vi "Cycle_Diag_Table_Read_TL24.vi"(7 "ERD Data In":T3[](array[typedef]) {"ERD Number" format="%.0x"}, 11 "error in (no error)":errorcluster) -> (2 "Cycle Buffer Status":T2, 3 "Diag Cycle String Out":string[][](array[string]), 8 "Cycle  Diag Array Out":T1[](array[typedef]), 15 "error out":errorcluster)   [LabVIEW 2016]
uses:
  Common/LabVIEW GEA2 Toolkit/LabVIEW_GEA2_Toolkit.lvlibp/type defs/ERD Read Data Out.ctl
  type defs/Cycle_Diag_Buffer_Status.ctl
  type defs/Cycle_Diag.ctl
  Common/LabVIEW GEA2 Toolkit/LabVIEW_GEA2_Toolkit.lvlibp
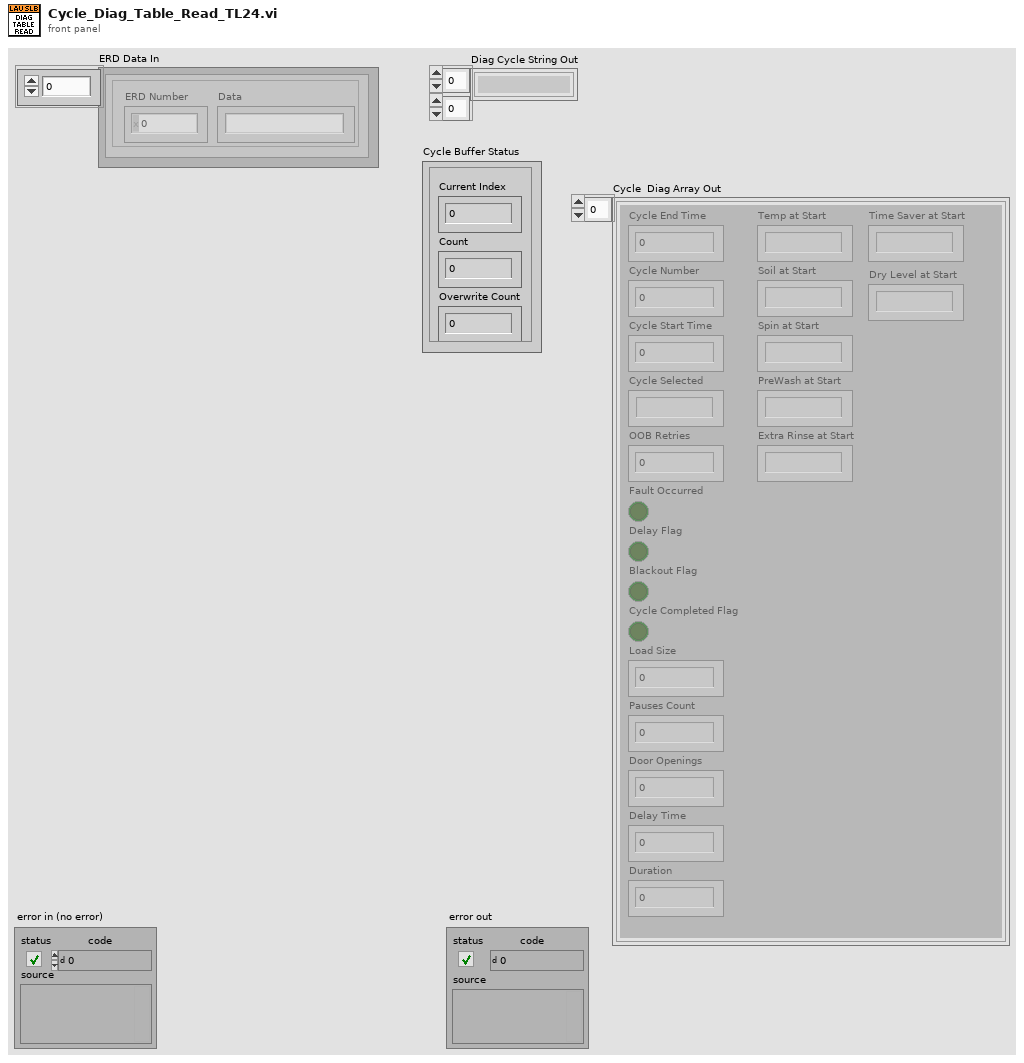
[diagram p1: front panel]
types:
  T1 = typedef "Cycle_Diag.ctl" = cluster{"Cycle End Time":u32, "Cycle Number":u32, "Cycle Start Time":u32, "OOB Retries":u8, "Temp at Start":string, "Soil at Start":string, "PreWash at Start":string, "Extra Rinse at Start":string, "Pauses Count":u8, "Fault Occurred":bool, "Delay Flag":bool, "Blackout Flag":bool, "Cycle Completed Flag":bool, "Time Saver at Start":string, "Load Size":u8, "Door Openings":u8, "Cycle Selected":string, "Spin at Start":string, "Delay Time":u16, "Duration":dbl, "Dry Level at Start":string}
  T2 = typedef "Cycle_Diag_Buffer_Status.ctl" = cluster{"Current Index":u16, "Count":u16, "Overwrite Count":u16}
  T3 = typedef "LabVIEW_GEA2_Toolkit.lvlibp/ERD Read Data Out.ctl" = cluster{"ERD Number":u16, "Data":string}
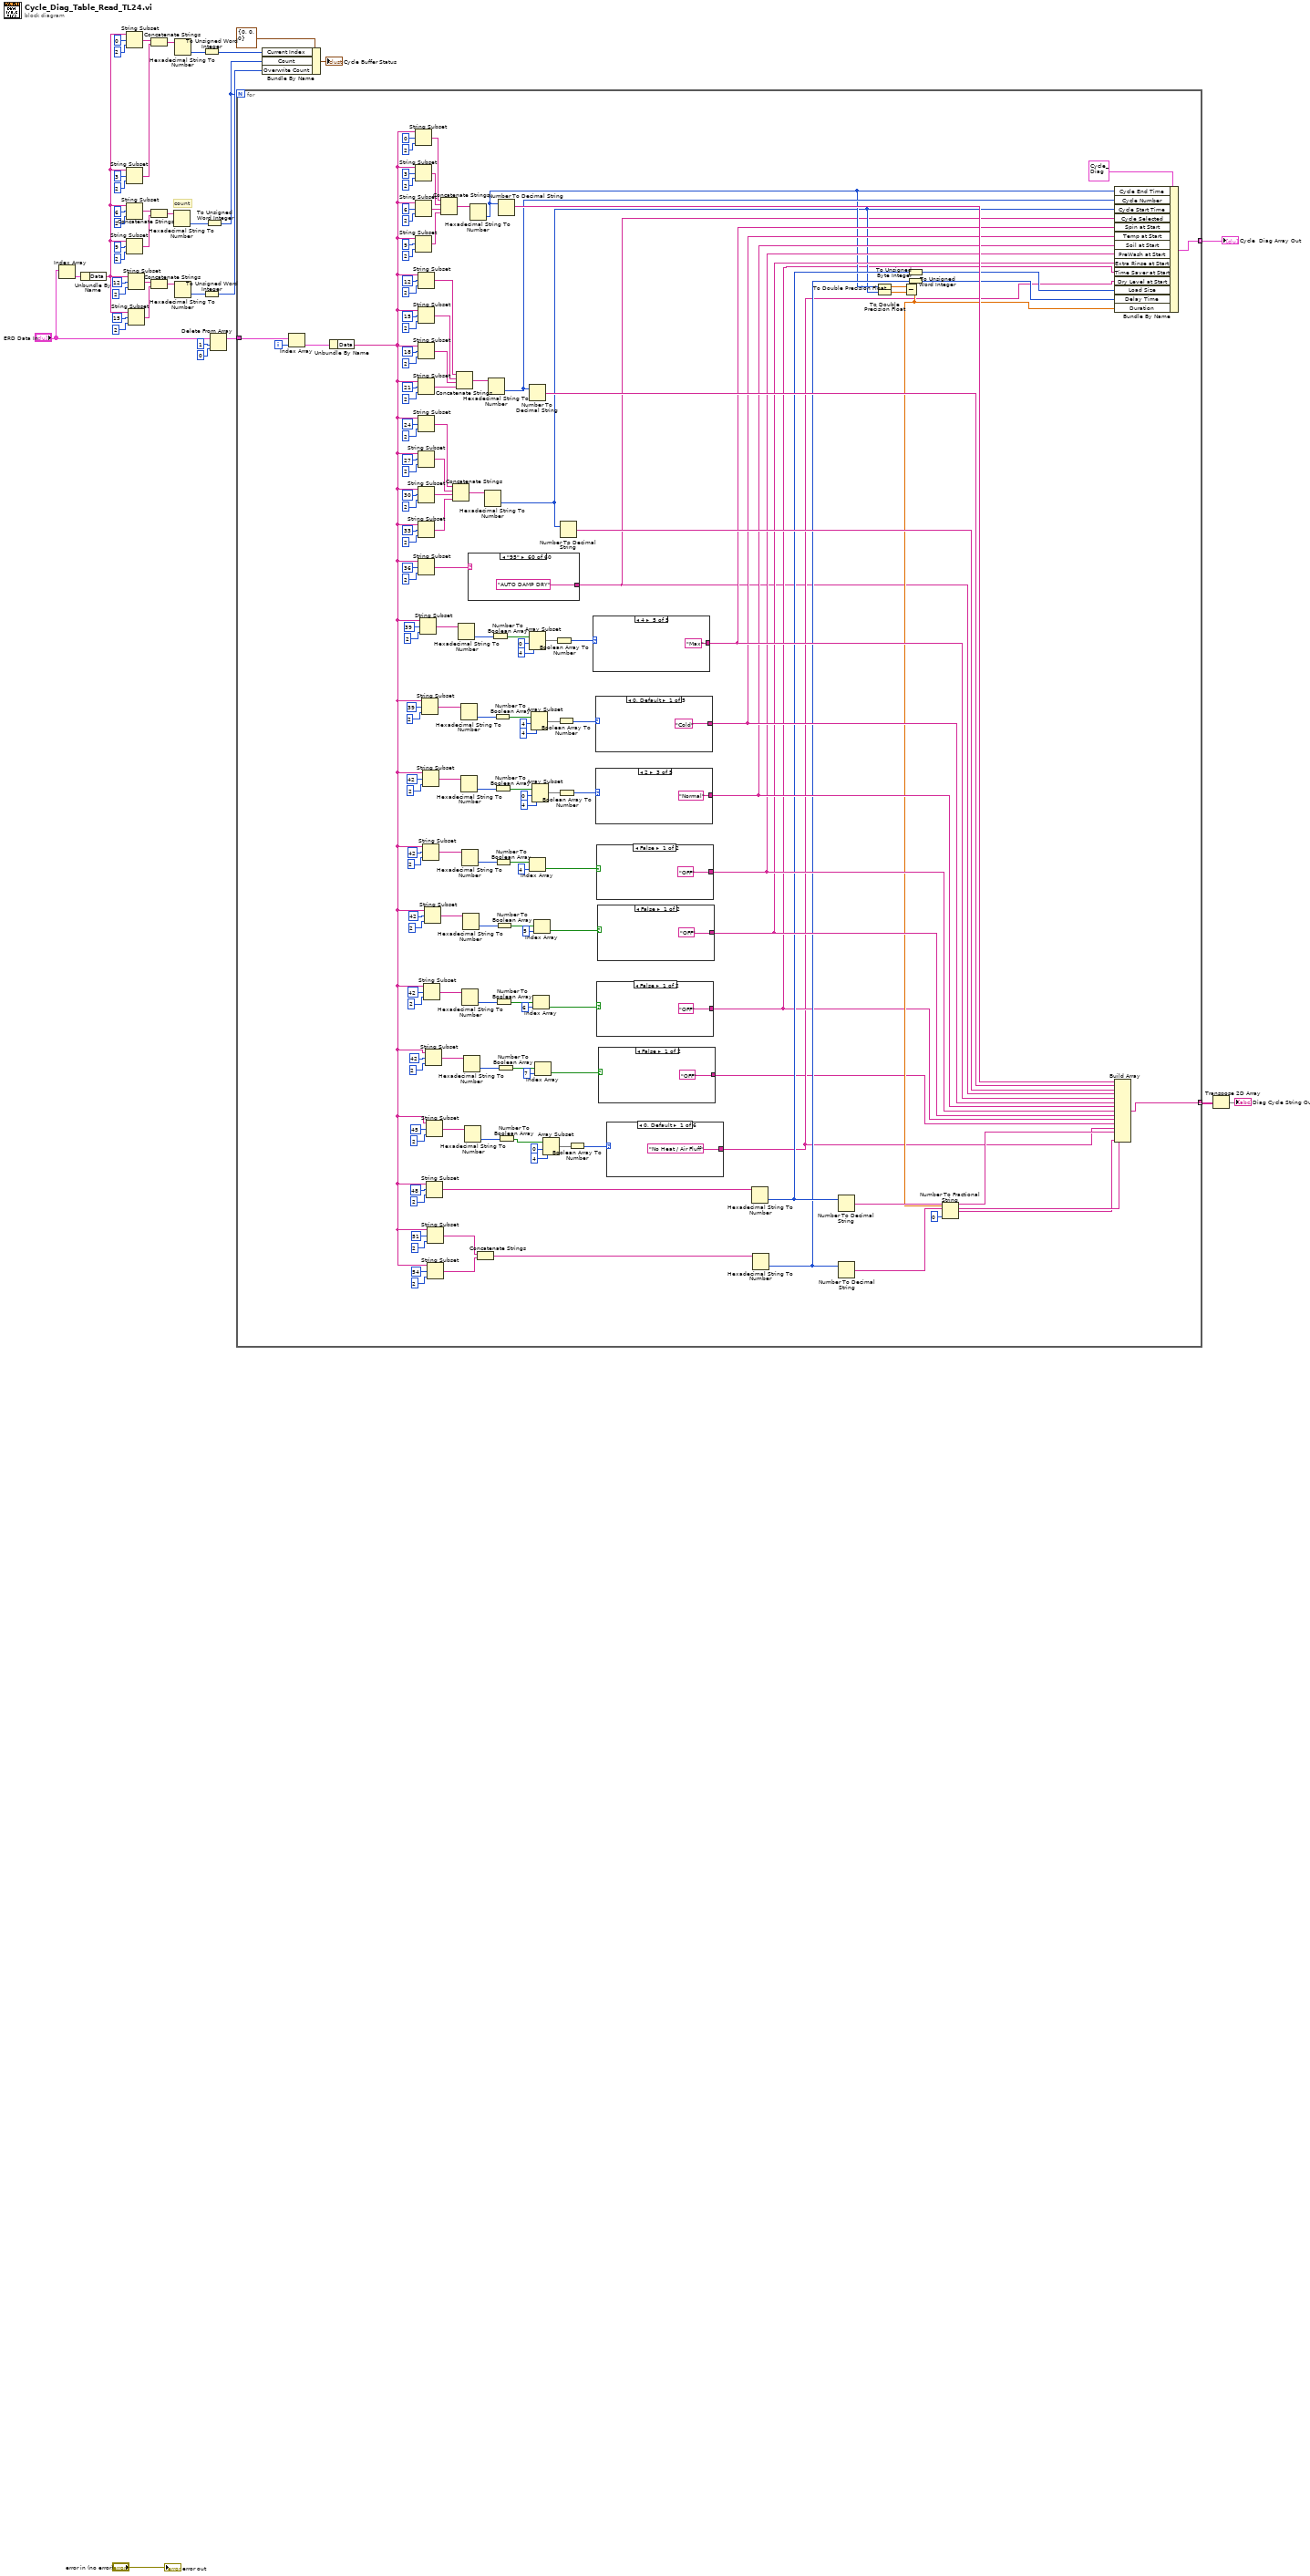
[diagram p0: block diagram]
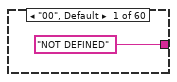
[diagram p2: hidden frame]
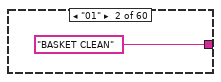
[diagram p3: hidden frame]
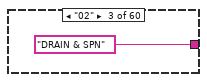
[diagram p4: hidden frame]
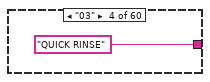
[diagram p5: hidden frame]
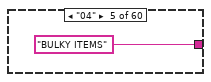
[diagram p6: hidden frame]
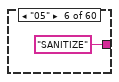
[diagram p7: hidden frame]
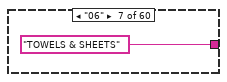
[diagram p8: hidden frame]
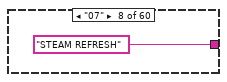
[diagram p9: hidden frame]
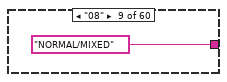
[diagram p10: hidden frame]
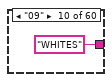
[diagram p11: hidden frame]
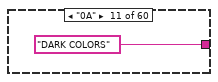
[diagram p12: hidden frame]
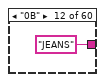
[diagram p13: hidden frame]
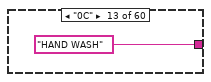
[diagram p14: hidden frame]
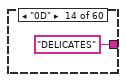
[diagram p15: hidden frame]
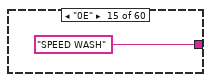
[diagram p16: hidden frame]
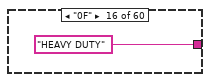
[diagram p17: hidden frame]
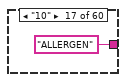
[diagram p18: hidden frame]
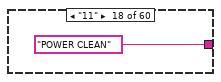
[diagram p19: hidden frame]
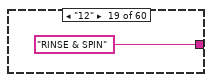
[diagram p20: hidden frame]
diagram:
  # "count"
  n1 = Index Array(array="ERD Data In") -> (element=w32:T3)  [unwired: 1 in]
  n2 = Unbundle By Name(w32) -> ("Data"=w12:string)
  n3 = String Subset(string=w12, offset (0)=0, length (rest)=2 ("length (rest)")) -> (substring=w21:string)
  n4 = String Subset(string=w12, offset (0)=3, length (rest)=2 ("length (rest)")) -> (substring=w22:string)
  n5 = String Subset(string=w12, offset (0)=6, length (rest)=2 ("length (rest)")) -> (substring=w36:string)
  n6 = String Subset(string=w12, offset (0)=9, length (rest)=2 ("length (rest)")) -> (substring=w35:string)
  n7 = String Subset(string=w12, offset (0)=12, length (rest)=2 ("length (rest)")) -> (substring=w23:string)
  n8 = String Subset(string=w12, offset (0)=15, length (rest)=2 ("length (rest)")) -> (substring=w24:string)
  n9 = Concatenate Strings(w21, w22) -> (w25:string)
  n10 = Concatenate Strings(w36, w35) -> (w34:string)
  n11 = Concatenate Strings(w23, w24) -> (w26:string)
  n12 = Hexadecimal String To Number(string=w34) -> (number=w33:u32)  [unwired: 2 in, 1 out]
  n13 = Hexadecimal String To Number(string=w25) -> (number=w27:u32)  [unwired: 2 in, 1 out]
  n14 = Hexadecimal String To Number(string=w26) -> (number=w28:u32)  [unwired: 2 in, 1 out]
  n15 = To Unsigned Word Integer(number=w27) -> (unsigned 16bit integer=w29:u16)
  n16 = To Unsigned Word Integer(number=w28) -> (unsigned 16bit integer=w30:u16)
  n17 = To Unsigned Word Integer(number=w33) -> (unsigned 16bit integer=w11:u16)
  n18 = Delete From Array(array="ERD Data In", length=1, index=0) -> (array with subset deleted=w8:T3[])  [unwired: 1 out]
  n19 = for {
    N: w11 -> [_]
    tunnel: w8 -> [w147]
    tunnel: [w144] -> w4 mode=indexing
    tunnel: [w143] -> w3 mode=indexing
    i -> [w146]
    n20 = Index Array(array=w147, index=w146) -> (element=w145:T3)
    n21 = Unbundle By Name(w145) -> ("Data"=w43:string)
    n22 = String Subset(string=w43, offset (0)=0, length (rest)=2 ("length (rest)")) -> (substring=w162:string)
    n23 = String Subset(string=w43, offset (0)=3, length (rest)=2 ("length (rest)")) -> (substring=w161:string)
    n24 = String Subset(string=w43, offset (0)=6, length (rest)=2 ("length (rest)")) -> (substring=w160:string)
    n25 = String Subset(string=w43, offset (0)=9, length (rest)=2 ("length (rest)")) -> (substring=w159:string)
    n26 = String Subset(string=w43, offset (0)=12, length (rest)=2 ("length (rest)")) -> (substring=w157:string)
    n27 = String Subset(string=w43, offset (0)=15, length (rest)=2 ("length (rest)")) -> (substring=w156:string)
    n28 = String Subset(string=w43, offset (0)=18, length (rest)=2 ("length (rest)")) -> (substring=w155:string)
    n29 = String Subset(string=w43, offset (0)=21, length (rest)=2 ("length (rest)")) -> (substring=w154:string)
    n30 = String Subset(string=w43, offset (0)=24, length (rest)=2 ("length (rest)")) -> (substring=w152:string)
    n31 = String Subset(string=w43, offset (0)=27, length (rest)=2 ("length (rest)")) -> (substring=w151:string)
    n32 = String Subset(string=w43, offset (0)=30, length (rest)=2 ("length (rest)")) -> (substring=w150:string)
    n33 = String Subset(string=w43, offset (0)=33, length (rest)=2 ("length (rest)")) -> (substring=w149:string)
    n34 = String Subset(string=w43, offset (0)=36, length (rest)=2 ("length (rest)")) -> (substring=w41:string)
    n35 = String Subset(string=w43, offset (0)=39, length (rest)=2 ("length (rest)")) -> (substring=w135:string)
    n36 = String Subset(string=w43, offset (0)=39, length (rest)=2 ("length (rest)")) -> (substring=w121:string)
    n37 = String Subset(string=w43, offset (0)=42, length (rest)=2 ("length (rest)")) -> (substring=w115:string)
    n38 = String Subset(string=w43, offset (0)=42, length (rest)=2 ("length (rest)")) -> (substring=w106:string)
    n39 = String Subset(string=w43, offset (0)=42, length (rest)=2 ("length (rest)")) -> (substring=w66:string)
    n40 = String Subset(string=w43, offset (0)=42, length (rest)=2 ("length (rest)")) -> (substring=w100:string)
    n41 = String Subset(string=w43, offset (0)=42, length (rest)=2 ("length (rest)")) -> (substring=w46:string)
    n42 = String Subset(string=w43, offset (0)=45, length (rest)=2 ("length (rest)")) -> (substring=w59:string)
    n43 = String Subset(string=w43, offset (0)=48, length (rest)=2 ("length (rest)")) -> (substring=w91:string)
    n44 = String Subset(string=w43, offset (0)=51, length (rest)=2 ("length (rest)")) -> (substring=w82:string)
    n45 = String Subset(string=w43, offset (0)=54, length (rest)=2 ("length (rest)")) -> (substring=w81:string)
    n46 = Concatenate Strings(w162, w161, w160, w159) -> (w158:string)
    n47 = Concatenate Strings(w152, w151, w150, w149) -> (w148:string)
    n48 = Concatenate Strings(w157, w156, w155, w154) -> (w153:string)
    n49 = Hexadecimal String To Number(string=w135) -> (number=w134:u32)  [unwired: 2 in, 1 out]
    n50 = Hexadecimal String To Number(string=w121) -> (number=w122:u32)  [unwired: 2 in, 1 out]
    n51 = Hexadecimal String To Number(string=w115) -> (number=w114:u32)  [unwired: 2 in, 1 out]
    n52 = Hexadecimal String To Number(string=w106) -> (number=w107:u32)  [unwired: 2 in, 1 out]
    n53 = Hexadecimal String To Number(string=w66) -> (number=w65:u32)  [unwired: 2 in, 1 out]
    n54 = Hexadecimal String To Number(string=w100) -> (number=w99:u32)  [unwired: 2 in, 1 out]
    n55 = Hexadecimal String To Number(string=w46) -> (number=w47:u32)  [unwired: 2 in, 1 out]
    n56 = Hexadecimal String To Number(string=w59) -> (number=w58:u32)  [unwired: 2 in, 1 out]
    n57 = case shown="\"95\"" w41 {
      tunnel: ["NOT DEFINED" "BASKET CLEAN" "DRAIN & SPN" "QUICK RINSE" "BULKY ITEMS" "SANITIZE" "TOWELS & SHEETS" "STEAM REFRESH" "NORMAL/MIXED" "WHITES" "DARK COLORS" "JEANS" "HAND WASH" "DELICATES" "SPEED WASH" "HEAVY DUTY" "ALLERGEN" "POWER CLEAN" "RINSE & SPIN" "SINGLE ITEM" "COLORS" "COLD WASH" "WATER STATION" "TUB CLEAN" "CASUALS W/ STEAM" "STAIN WASH W/ STEAM" "DEEP CLEAN" "BULKY BEDDING" "NORMAL" "QUICK WASH" "SANITIZE W/ OXI" "SELF CLEAN" "TOWELS" "SOAK" "WOOL" "ULTRA FRESH VENT" "SANITIZE & ALLERGEN" "SPIN ONLY" "COTTONS" "EASY CARE" "ACTIVE WEAR" "TIMED DRY" "DEWRINKLE" "AIR FLUFF" "STEAM REFRESH" "STEAM DEWRINKLE" "SPEED DRY" "MIXED" "QUICK DRY" "CASUALS" "WARM UP" "ENERGY SAVER" "ANTIBACTERIAL" "RACK DRY" "BABY CARE" "AUTO DRY" "AUTO EXTRA DRY" "PERM PRESS" "WASHER LINK" "AUTO DAMP DRY"] -> w40
      frame "00", Default {
      }
      frame "01" {
      }
      frame "02" {
      }
      frame "03" {
      }
      frame "04" {
      }
      frame "05" {
      }
      frame "06" {
      }
      frame "07" {
      }
      frame "08" {
      }
      frame "09" {
      }
      frame "0A" {
      }
      frame "0B" {
      }
      frame "0C" {
      }
      frame "0D" {
      }
      frame "0E" {
      }
      frame "0F" {
      }
      frame "10" {
      }
      frame "11" {
      }
      frame "12" {
      }
      frame "13" {
      }
      frame "14" {
      }
      frame "15" {
      }
      frame "16" {
      }
      frame "17" {
      }
      frame "18" {
      }
      frame "19" {
      }
      frame "1A" {
      }
      frame "1B" {
      }
      frame "1C" {
      }
      frame "1D" {
      }
      frame "1E" {
      }
      frame "1F" {
      }
      frame "20" {
      }
      frame "21" {
      }
      frame "22" {
      }
      frame "23" {
      }
      frame "24" {
      }
      frame "25" {
      }
      frame "80" {
      }
      frame "81" {
      }
      frame "82" {
      }
      frame "83" {
      }
      frame "84" {
      }
      frame "85" {
      }
      frame "86" {
      }
      frame "87" {
      }
      frame "88" {
      }
      frame "89" {
      }
      frame "8A" {
      }
      frame "8B" {
      }
      frame "8C" {
      }
      frame "8D" {
      }
      frame "8E" {
      }
      frame "8F" {
      }
      frame "90" {
      }
      frame "91" {
      }
      frame "92" {
      }
      frame "93" {
      }
      frame "94" {
      }
      frame "95" {
      }
    }
    n58 = Hexadecimal String To Number(string=w158) -> (number=w76:u32)  [unwired: 2 in, 1 out]
    n59 = Concatenate Strings(w82, w81) -> (w80:string)
    n60 = Hexadecimal String To Number(string=w148) -> (number=w75:u32)  [unwired: 2 in, 1 out]
    n61 = Hexadecimal String To Number(string=w153) -> (number=w139:u32)  [unwired: 2 in, 1 out]
    n62 = Number To Boolean Array(number=w134) -> (Boolean array=w133:bool[])
    n63 = Number To Boolean Array(number=w122) -> (Boolean array=w123:bool[])
    n64 = Number To Boolean Array(number=w114) -> (Boolean array=w113:bool[])
    n65 = Number To Boolean Array(number=w107) -> (Boolean array=w95:bool[])
    n66 = Number To Boolean Array(number=w65) -> (Boolean array=w64:bool[])
    n67 = Number To Boolean Array(number=w99) -> (Boolean array=w98:bool[])
    n68 = Number To Boolean Array(number=w47) -> (Boolean array=w48:bool[])
    n69 = Number To Decimal String(number=w76) -> (decimal integer string=w141:string)  [unwired: 1 in]
    n70 = Number To Boolean Array(number=w58) -> (Boolean array=w53:bool[])
    n71 = Number To Decimal String(number=w139) -> (decimal integer string=w140:string)  [unwired: 1 in]
    n72 = Array Subset(array=w133, index=0, length=4) -> (w130:bool[])
    n73 = Index Array(array=w95, index=4) -> (element=w94:bool)
    n74 = Array Subset(array=w123, index=4, length=4) -> (w126:bool[])
    n75 = Array Subset(array=w113, index=0, length=4) -> (w110:bool[])
    n76 = Index Array(array=w64, index=6) -> (element=w62:bool)
    n77 = Index Array(array=w98, index=5) -> (element=w93:bool)
    n78 = Index Array(array=w48, index=7) -> (element=w50:bool)
    n79 = Array Subset(array=w53, index=0, length=4) -> (w55:bool[])
    n80 = Boolean Array To Number(Boolean array=w130) -> (number=w129:u32)
    n81 = Boolean Array To Number(Boolean array=w126) -> (number=w127:u32)
    n82 = Boolean Array To Number(Boolean array=w110) -> (number=w109:u32)
    n83 = Number To Decimal String(number=w75) -> (decimal integer string=w138:string)  [unwired: 1 in]
    n84 = Boolean Array To Number(Boolean array=w55) -> (number=w54:u32)
    n85 = case shown="4" w129 {
      tunnel: ["No Spin" "Low" "Medium" "High" "Max"] -> w128
      frame 0, Default {
      }
      frame 1 {
      }
      frame 2 {
      }
      frame 3 {
      }
      frame 4 {
      }
    }
    n86 = case shown="0, Default" w127 {
      tunnel: ["Cold" "Cool" "Warm" "Hot" "Extra Hot"] -> w118
      frame 0, Default {
      }
      frame 1 {
      }
      frame 2 {
      }
      frame 3 {
      }
      frame 4 {
      }
    }
    n87 = case shown="2" w109 {
      tunnel: ["Extra Light" "Light" "Normal" "Heavy" "Extra Heavy"] -> w108
      frame 0, Default {
      }
      frame 1 {
      }
      frame 2 {
      }
      frame 3 {
      }
      frame 4 {
      }
    }
    n88 = case shown="False" w94 {
      tunnel: ["OFF" "ON"] -> w103
      frame False {
      }
      frame True {
      }
    }
    n89 = case shown="False" w62 {
      tunnel: ["OFF" "ON"] -> w52
      frame False {
      }
      frame True {
      }
    }
    n90 = case shown="False" w93 {
      tunnel: ["OFF" "ON"] -> w92
      frame False {
      }
      frame True {
      }
    }
    n91 = case shown="False" w50 {
      tunnel: ["OFF" "ON"] -> w42
      frame False {
      }
      frame True {
      }
    }
    n92 = case shown="0, Default" w54 {
      tunnel: ["No Heat / Air Fluff" "Extra Low" "Low" "Medium" "High" "Off"] -> w51
      frame 0, Default {
      }
      frame 1 {
      }
      frame 2 {
      }
      frame 3 {
      }
      frame 4 {
      }
      frame 5 {
      }
    }
    n93 = Hexadecimal String To Number(string=w91) -> (number=w87:u32)  [unwired: 2 in, 1 out]
    n94 = Hexadecimal String To Number(string=w80) -> (number=w78:u32)  [unwired: 2 in, 1 out]
    n95 = Number To Decimal String(number=w87) -> (decimal integer string=w88:string)  [unwired: 1 in]
    n96 = Number To Decimal String(number=w78) -> (decimal integer string=w79:string)  [unwired: 1 in]
    n97 = To Double Precision Float(number=w76) -> (double precision float=w74:dbl)
    n98 = To Double Precision Float(number=w75) -> (double precision float=w73:dbl)
    n99 = Subtract(x=w74, y=w73) -> (x-y=w71:dbl)
    n100 = To Unsigned Byte Integer(number=w87) -> (unsigned 8bit integer=w69:u8)
    n101 = To Unsigned Word Integer(number=w78) -> (unsigned 16bit integer=w77:u16)
    n102 = Number To Fractional String(number=w71, precision (6)=i16 0) -> (F-format string=w72:string)  [unwired: 2 in]
    n103 = Bundle By Name(cluster=T1 {"Cycle End Time"=0, "Cycle Number"=0, "Cycle Start Time"=0, "OOB Retries"=0, "Temp at Start"="", "Soil at Start"="", "PreWash at Start"="", "Extra Rinse at Start"="", "Pauses Count"=0, "Fault Occurred"=FALSE, "Delay Flag"=FALSE, "Blackout Flag"=FALSE, "Cycle Completed Flag"=FALSE, "Time Saver at Start"="", "Load Size"=0, "Door Openings"=0, "Cycle Selected"="", "Spin at Start"="", "Delay Time"=0, "Duration"=0.0, "Dry Level at Start"=""} ("Cycle History Diagnostics"), "Cycle End Time"=w76, "Cycle Number"=w139, "Cycle Start Time"=w75, "Cycle Selected"=w40, "Spin at Start"=w128, "Temp at Start"=w118, "Soil at Start"=w108, "PreWash at Start"=w103, "Extra Rinse at Start"=w92, "Time Saver at Start"=w52, "Dry Level at Start"=w51, "Load Size"=w69, "Delay Time"=w77, "Duration"=w71) -> (w144:T1)
    n104 = Build Array(w141, w140, w138, w40, w128, w118, w108, w103, w92, w52, w42, w51, w88, w79, w72) -> (w143:string[])
  }
  "Cycle  Diag Array Out" <- w4
  n105 = Bundle By Name(cluster=T2 {"Current Index"=0, "Count"=0, "Overwrite Count"=0} ("Cycle Buffer Status"), "Current Index"=w29, "Count"=w11, "Overwrite Count"=w30) -> (→"Cycle Buffer Status":T2)
  n106 = Transpose 2D Array(2D array=w3) -> (transposed array=→"Diag Cycle String Out":string[][])
  "error out" <- "error in (no error)"
